vi "Init.vi"(7 "TableRef":refnum<vi>, 8 "error in (no error)":errorcluster, 10 "show":T1) -> (0 "error out":errorcluster, 2 "Size":T4)   [LabVIEW 2021, in "RocketPlot.lvlib" / "TipTablePanel.lvclass"]
uses:
  TipTablePanel.lvclass
  <vilib>/Utility/miscctls.llb/LVBoundsTypeDef.ctl
  new tip instructions.ctl
  cell cache.ctl
  colors.ctl
  <vilib>/Utility/miscctls.llb/LVRowAndColumnTypeDef.ctl
  <vilib>/picture/picture.llb/Get Text Rect.vi
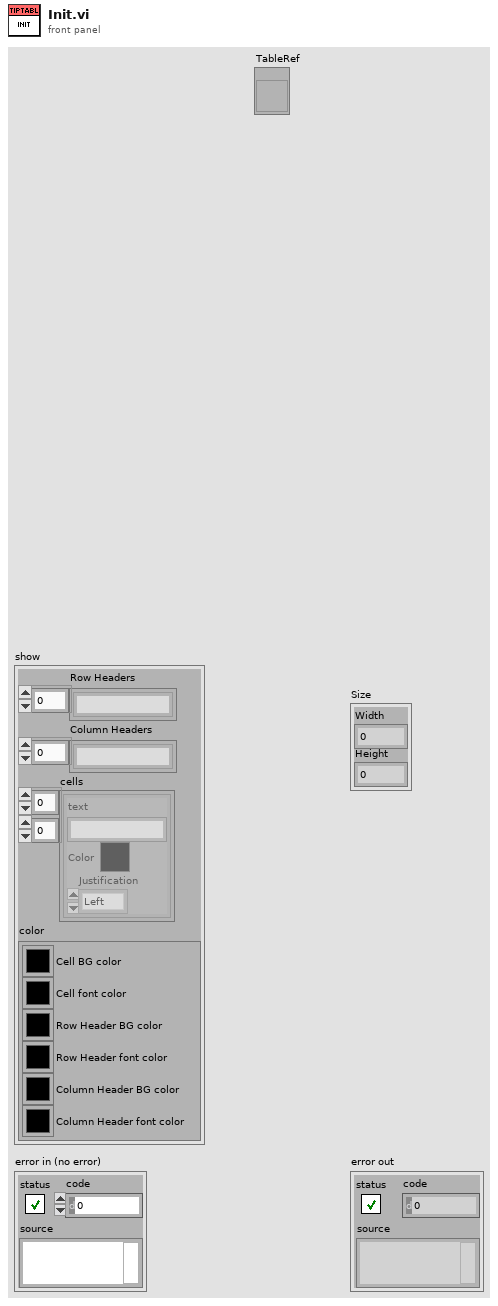
[diagram p1: front panel]
types:
  T1 = typedef "RocketPlot.lvlib/TipTablePanel.lvclass/new tip instructions.ctl" = cluster{"Row Headers":string[], "Column Headers":string[], "cells":T2[][], "color":T3}
  T2 = typedef "RocketPlot.lvlib/TipTablePanel.lvclass/cell cache.ctl" = cluster{"text":string, "Color":u32, "Justification":enum16{"Left", "Center", "Right"}}
  T3 = typedef "RocketPlot.lvlib/TipTablePanel.lvclass/colors.ctl" = cluster{"Cell BG color":u32, "Cell font color":u32, "Row Header BG color":u32, "Row Header font color":u32, "Column Header BG color":u32, "Column Header font color":u32}
  T4 = typedef "LVBoundsTypeDef.ctl" = cluster{"Width":u32, "Height":u32}
  T5 = typedef "LVRowAndColumnTypeDef.ctl" = cluster{"Row":i32, "Column":i32}
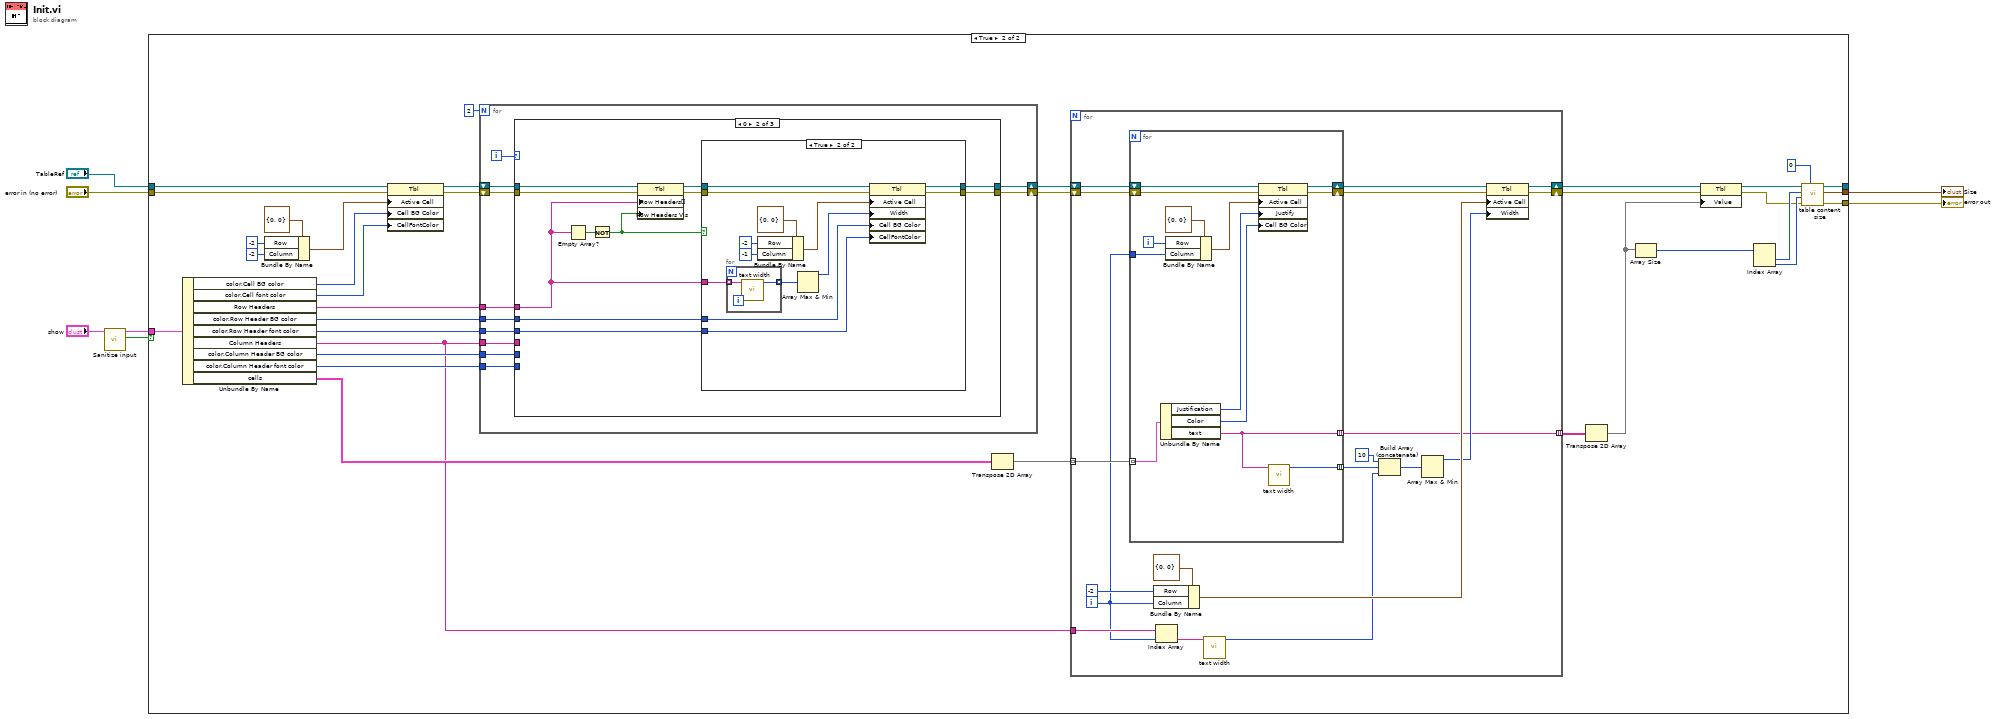
[diagram p0: block diagram]
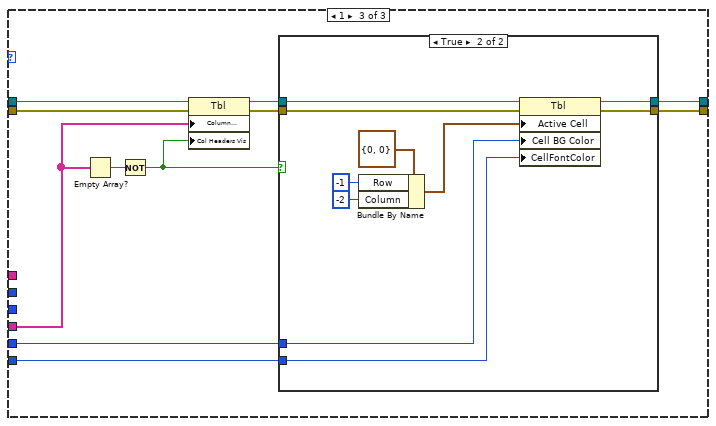
[diagram p5: hidden frame]
diagram:
  n1 = call "Sanitize input.vi"("TipTable"="show") -> ("valid?"=w2:bool, "TipTable"=w3:T1)  [unwired: 9 in]
  n2 = case shown="True" w2 {
    tunnel: "error in (no error)" -> [w9 w44]
    tunnel: [_ w43] -> w6
    tunnel: [w9 w42] -> w1
    tunnel: "TableRef" -> [w8 w41]
    tunnel: [w8 w40] -> _
    tunnel: w3 -> [_ w39]
    frame False {
    }
    frame True {
      n3 = Unbundle By Name(w39) -> ("color.Cell BG color"=w28:u32, "color.Cell font color"=w29:u32, "Row Headers"=w22:string[], "color.Row Header BG color"=w33:u32, "color.Row Header font color"=w32:u32, "Column Headers"=w17:string[], "color.Column Header BG color"=w20:u32, "color.Column Header font color"=w19:u32, "cells"=w21:T2[][])
      n4 = Bundle By Name(cluster=T5 {"Row"=0, "Column"=0} ("Active Cell:Active Cell"), "Row"=-2, "Column"=-2) -> (w34:T5)
      n5 = property class="Tbl"(reference=w41, error in=w44, "Active Cell"=w34, "Cell BG Color"=w28, "CellFontColor"=w29) -> (reference out=w27:refnum<vi>, error out=w26:errorcluster)
      n6 = for {
        N: 2 -> [_]
        tunnel: w33 -> [w55]
        tunnel: w32 -> [w54]
        tunnel: w22 -> [w49]
        shift-right: [w53] -> w31
        shift-left: w27 -> [w51]
        shift-right: [w52] -> w30
        shift-left: w26 -> [w50]
        tunnel: w17 -> [w47]
        tunnel: w20 -> [w46]
        tunnel: w19 -> [w45]
        i -> [w48]
        n7 = case shown="0" w48 {
          tunnel: w55 -> [_ w68 _]
          tunnel: w54 -> [_ w67 _]
          tunnel: [w57 w66 w96] -> w53
          tunnel: [w56 w65 w95] -> w52
          tunnel: w51 -> [w57 w61 w91]
          tunnel: w50 -> [w56 w60 w90]
          tunnel: w49 -> [_ w58 _]
          tunnel: w47 -> [_ _ w88]
          tunnel: w46 -> [_ _ w87]
          tunnel: w45 -> [_ _ w86]
          frame Default {
          }
          frame 0 {
            n8 = Empty Array?(array=w58) -> (empty?=w64:bool)
            n9 = Not(x=w64) -> (.not. x?=w59:bool)
            n10 = property class="Tbl"(reference=w61, error in=w60, "Row Headers[]"=w58, "Row Headers Vis"=w59) -> (reference out=w63:refnum<vi>, error out=w62:errorcluster)
            n11 = case shown="True" w59 {
              tunnel: w63 -> [w70 w83]
              tunnel: w68 -> [_ w78]
              tunnel: w67 -> [_ w77]
              tunnel: [w70 w76] -> w66
              tunnel: w62 -> [w69 w75]
              tunnel: [w69 w74] -> w65
              tunnel: w58 -> [_ w73]
              frame False {
              }
              frame True {
                n12 = for {
                  tunnel: w73 -> [w85] mode=indexing
                  tunnel: [w84] -> w72 mode=indexing
                  n13 = call "text width.vi"("text"=w85) -> ("Min Cell Width"=w84:u32)  [unwired: 10 in]
                }
                n14 = Bundle By Name(cluster=T5 {"Row"=0, "Column"=0} ("Active Cell:Active Cell"), "Row"=-2, "Column"=-1) -> (w79:T5)
                n15 = Array Max & Min(array=w72) -> (max value=w71:u32)  [unwired: 3 out]
                n16 = property class="Tbl"(reference=w83, error in=w75, "Active Cell"=w79, "Width"=w71, "Cell BG Color"=w78, "CellFontColor"=w77) -> (reference out=w76:refnum<vi>, error out=w74:errorcluster)
              }
            }
          }
          frame 1 {
            n17 = Empty Array?(array=w88) -> (empty?=w94:bool)
            n18 = Not(x=w94) -> (.not. x?=w89:bool)
            n19 = property class="Tbl"(reference=w91, error in=w90, "Column Headers[]"=w88, "Col Headers Vis"=w89) -> (reference out=w93:refnum<vi>, error out=w92:errorcluster)
            n20 = case shown="True" w89 {
              tunnel: w93 -> [w98 w108]
              tunnel: w87 -> [_ w103]
              tunnel: w86 -> [_ w102]
              tunnel: [w98 w101] -> w96
              tunnel: w92 -> [w97 w100]
              tunnel: [w97 w99] -> w95
              frame False {
              }
              frame True {
                n21 = Bundle By Name(cluster=T5 {"Row"=0, "Column"=0} ("Active Cell:Active Cell"), "Row"=-1, "Column"=-2) -> (w104:T5)
                n22 = property class="Tbl"(reference=w108, error in=w100, "Active Cell"=w104, "Cell BG Color"=w103, "CellFontColor"=w102) -> (reference out=w101:refnum<vi>, error out=w99:errorcluster)
              }
            }
          }
        }
      }
      n23 = Transpose 2D Array(2D array=w21) -> (transposed array=w38:T2[][])
      n24 = for {
        tunnel: w38 -> [w127] mode=indexing
        shift-right: [w120] -> w15
        shift-left: w31 -> [w118]
        shift-right: [w119] -> w14
        shift-left: w30 -> [w117]
        tunnel: w17 -> [w113]
        tunnel: [w111] -> w13 mode=indexing
        i -> [w112]
        n25 = for {
          tunnel: w127 -> [w132] mode=indexing
          tunnel: [w128] -> w123 mode=indexing
          shift-right: [w138] -> w116
          shift-left: w118 -> [w140]
          shift-right: [w137] -> w115
          shift-left: w117 -> [w139]
          tunnel: w112 -> [w134]
          tunnel: [w129] -> w111 mode=indexing
          i -> [w133]
          n26 = Unbundle By Name(w132) -> ("Justification"=w131:enum16{"Left", "Center", "Right"}, "Color"=w130:u32, "text"=w129:string)
          n27 = Bundle By Name(cluster=T5 {"Row"=0, "Column"=0} ("Active Cell:Active Cell"), "Row"=w133, "Column"=w134) -> (w135:T5)
          n28 = property class="Tbl"(reference=w140, error in=w139, "Active Cell"=w135, "Justify"=w131, "Cell BG Color"=w130) -> (reference out=w138:refnum<vi>, error out=w137:errorcluster)
          n29 = call "text width.vi"("text"=w129) -> ("Min Cell Width"=w128:u32)  [unwired: 10 in]
        }
        n30 = Bundle By Name(cluster=T5 {"Row"=0, "Column"=0} ("Active Cell:Active Cell"), "Row"=-2, "Column"=w112) -> (w124:T5)
        n31 = Index Array(array=w113, index=w112) -> (element=w110:string)
        n32 = call "text width.vi"("text"=w110) -> ("Min Cell Width"=w109:u32)  [unwired: 10 in]
        n33 = Build Array (concatenate)(u32 10 ("Min Cell Width"), w123, w109) -> (w121:u32[])
        n34 = Array Max & Min(array=w121) -> (max value=w114:u32)  [unwired: 3 out]
        n35 = property class="Tbl"(reference=w116, error in=w115, "Active Cell"=w124, "Width"=w114) -> (reference out=w120:refnum<vi>, error out=w119:errorcluster)
      }
      n36 = Transpose 2D Array(2D array=w13) -> (transposed array=w12:string[][])
      n37 = Array Size(array=w12) -> (size(s)=w25:i32[])
      n38 = property class="Tbl"(reference=w15, error in=w14, "Value"=w12) -> (reference out=w11:refnum<vi>, error out=w10:errorcluster)
      n39 = Index Array(array=w25) -> (element #1=w24:i32, element #2=w23:i32)  [unwired: 2 in]
      n40 = call "table content size.vi"("border (0px)"=0, "error in (no error)"=w10, "#columns"=w23, "#rows"=w24, "table"=w11) -> ("error out"=w42:errorcluster, "Size"=w43:T4, "table"=w40:refnum<vi>)  [unwired: 4 in]
    }
  }
  "error out" <- w1
  "Size" <- w6
